vi "Test_ExtCmd_Read.vi"() -> ()   [LabVIEW 2011]
uses:
  <vilib>/Instr/_visa.llb/VISA Configure Serial Port (Instr).vi
panel:
  out "Received":string
  in  "QUIT":bool
  in  "Excmd Baud rate":u32=38400
  in  "Excmd VRN":refnum<visa-resource-name>="COM8"
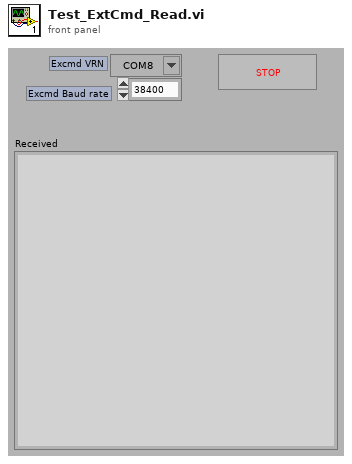
[diagram p1: front panel]
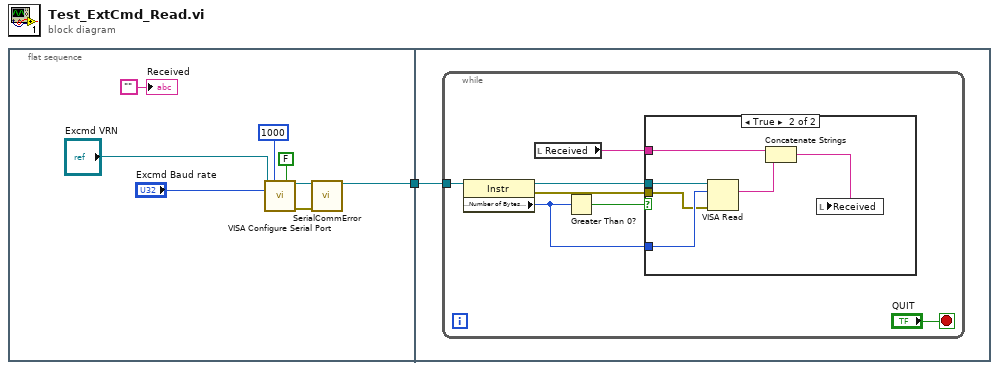
[diagram p0: block diagram]
diagram:
  n1 = flat-sequence {
    tunnel: [w3] -> w1
    tunnel: w1 -> [w10]
    frame #0 {
      n2 = call-poly "VISA Configure Serial Port"("VISA resource name"="Excmd VRN", "timeout (10sec)"=u32 1000, "Enable Termination\nChar (T)"=FALSE ("Enable Termination\nChar (T)"), "baud rate (9600)"="Excmd Baud rate") -> ("VISA resource name out"=w8:refnum<visa-resource-name>, "error out"=w9:errorcluster)  [unwired: 10 in]
      n3 = call "SerialCommError.vi"("VISA IN"=w8, "error IN"=w9) -> ("VISA OUT"=w3:refnum<visa-resource-name>)  [unwired: 11 in, 2 out]
      "Received" <- ""
    }
    frame #1 {
      n4 = while {
        tunnel: w10 -> [w16]
        stop <- "QUIT" stop-if-true
        n5 = property class="Instr"(reference=w16) -> (reference out=w13:refnum<visa-resource-name>, error out=w12:errorcluster, "Serial Settings:Number of Bytes at Serial Port"=w14:u32)  [unwired: 1 in]
        n6 = local read "Received"() -> (w11:string)
        n7 = Greater Than 0?(x=w14) -> (x > 0?=w15:bool)
        n8 = case shown="True" w15 {
          tunnel: w14 -> [_ w23]
          tunnel: w13 -> [_ w22]
          tunnel: w12 -> [_ w21]
          tunnel: w11 -> [_ w20]
          frame False {
          }
          frame True {
            n9 = VISA Read(VISA resource name=w22, byte count=w23, error in (no error)=w21) -> (read buffer=w19:string)  [unwired: 3 out]
            n10 = Concatenate Strings(w20, w19) -> (w18:string)
            n11 = local write "Received"(w18) -> ()
          }
        }
      }
    }
  }
